vi "Init.vi"(8 "error in (no error)":errorcluster caption="entrée d'erreur (pas d'erreur)", 11 "Process (Default) en entrée":refnum<class "Process (Default).lvclass">) -> (0 "error out":errorcluster caption="sortie d'erreur", 3 "Process (Default) en sortie":refnum<class "Process (Default).lvclass">)   [LabVIEW 2020, in "Library Instrument & Equipement.lvlib" / "Process (Default).lvclass"]
uses:
  Process (Default).lvclass
  Process (Default).lvclass/Process (Default).ctl
  Virtual Launch.vi
  Variable dispatch.vi
  Commun VI/Library Commun.lvlib
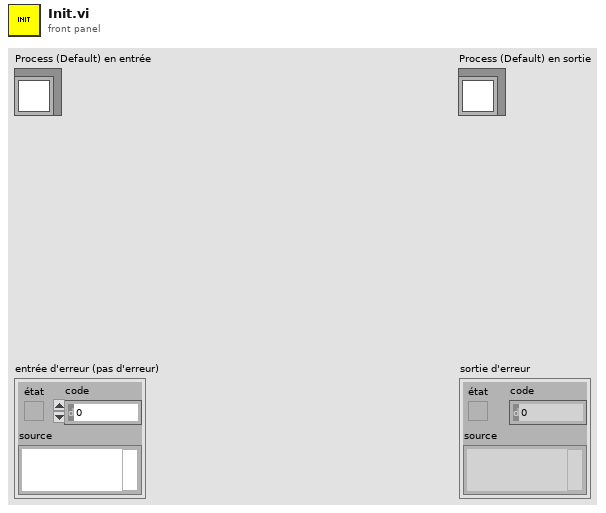
[diagram p1: front panel]
types:
  T1 = cluster{"Standard Output":string, "Process_is_Finish":bool}
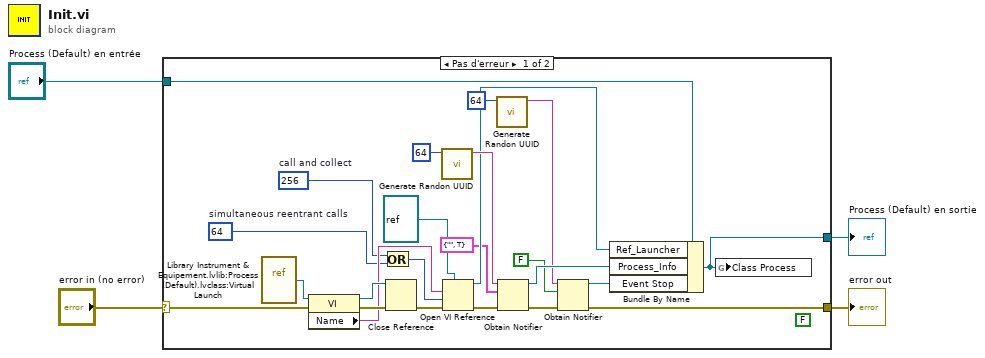
[diagram p0: block diagram]
diagram:
  n1 = case shown="Pas d'erreur" "error in (no error)" {
    selector: "error in (no error)" -> [w21 w30]
    tunnel: [w6 w30] -> w3
    tunnel: [w14 w29] -> w1
    tunnel: "Process (Default) en entrée" -> [w19 w29]
    frame No Error {
      (unwired) FALSE
      w17 = 64  # simultaneous reentrant calls
      w16 = 256  # call and collect
      n2 = vi-ref "Library Instrument & Equipement.lvlib:Process (Default).lvclass:Virtual Launch.vi"() -> (w26:refnum<vi>)
      n3 = property class="VI"(reference=w26, error in=w21) -> (reference out=w25:refnum<vi>, error out=w24:errorcluster, "Name"=w23:string)
      n4 = Or(x=w16, y=w17) -> (x .or. y?=w15:i32)
      n5 = Close Reference(reference=w25, error in (no error)=w24) -> (error out=w22:errorcluster)
      n6 = call "Generate Randon UUID.vi"("Taille"=64) -> ("chaîne"=w27:string)  [unwired: 10 in]
      n7 = Open VI Reference(type specifier VI Refnum (for type only)=refnum<vi> refnum ("spécificateur de type du refnum de VI (pour type seulement)"), vi path=w23, options=w15, error in (no error)=w22) -> (vi reference=w13:refnum<vi>, error out=w20:errorcluster)  [unwired: 2 in]
      n8 = call "Generate Randon UUID.vi"("Taille"=64) -> ("chaîne"=w9:string)  [unwired: 10 in]
      n9 = Obtain Notifier(name (unnamed)=w27, notification data type=T1 {"Standard Output"="", "Process_is_Finish"=TRUE}, error in (no error)=w20) -> (notifier out=w11:refnum<notifier>, error out=w7:errorcluster)  [unwired: 1 in, 1 out]
      n10 = Obtain Notifier(name (unnamed)=w9, notification data type=FALSE, error in (no error)=w7) -> (notifier out=w5:refnum<notifier>, error out=w6:errorcluster)  [unwired: 1 in, 1 out]
      n11 = Bundle By Name(cluster=w19, "Ref_Launcher"=w13, "Process_Info"=w11, "Event Stop"=w5) -> (w14:refnum<class "Process (Default).lvclass">)
      n12 = global write "Variable dispatch.vi" "Class Process"(w14) -> ()
    }
    frame Error {
    }
  }
  "error out" <- w3
  "Process (Default) en sortie" <- w1
